vi "Stop Core.vi"(10 "final error code":i32, 11 "DAM0404D in":refnum<class "DAM0404D.lvclass">) -> (3 "DAM0404D out":refnum<class "DAM0404D.lvclass">)   [LabVIEW 2016, in "DAM0404D.lvlib" / "DAM0404D.lvclass"]
doc: "(<B>Filename</B>: Actor Framework.lvlib:Actor.lvclass:Stop Core.vi)\n\nDefines what the actor does before it stops. Use the <B>final error code</B> input to determine whether the actor shut down in response to an error.\n\nBy default, this method does nothing. A descendant class may override it to define behavior, such as shutting down any processes the actor initiated in its override of the Actor Core method."
uses:
  DAM0404D.lvclass
  <vilib>/ActorFramework/Actor/Actor.lvclass
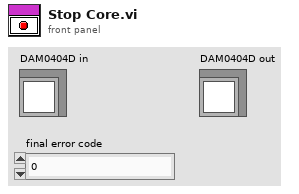
[diagram p1: front panel]
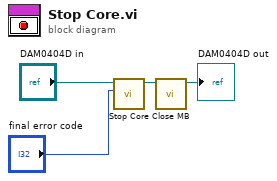
[diagram p0: block diagram]
diagram:
  n1 = call-parent "Stop Core.vi"("final error code"="final error code", "Actor in"="DAM0404D in") -> ("Actor out"=w2:refnum<class "DAM0404D.lvclass">)  [unwired: 9 in]
  n2 = call "Close MB.vi"("DAM0404D in"=w2) -> ("DAM0404D out"=→"DAM0404D out":refnum<class "DAM0404D.lvclass">)  [unwired: 9 in, 1 out]
